vi "Create Missing Source Folders.vi"(8 "error in":errorcluster, 9 "Install Root":string, 10 "Source Root":string, 11 "All Install Folders":path[](array[path])) -> (0 "error out":errorcluster, 1 "Install Root":string, 2 "Source Root":string)   [LabVIEW 2011, in "LVH-Build-Tools.lvlib"]
doc: "This VI creates folders in the source directory to match the folder hierarchy in the install directory."
uses:
  LVH-Build-Tools.lvlib
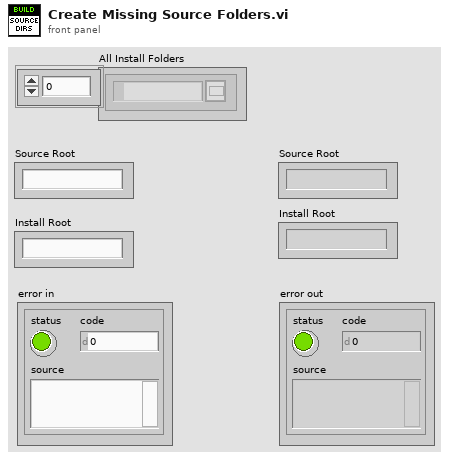
[diagram p1: front panel]
types:
  T1 = typedef "LVH-Build-Tools.lvlib/Configuration.ctl" = cluster{"Source Root":string, "Install Root":string, "Components":string[], "Ignore":string[]}
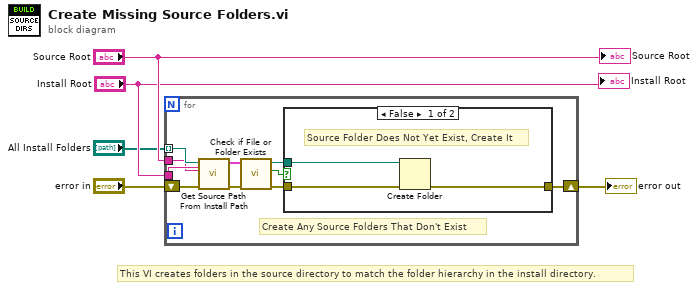
[diagram p0: block diagram]
diagram:
  # "This VI creates folders in the source directory to match the folder hierarchy in the install directory."
  n1 = for {
    tunnel: "All Install Folders" -> [w10] mode=indexing
    shift-right: [w12] -> w3
    shift-left: "error in" -> [w8]
    tunnel: "Install Root" -> [w7]
    tunnel: "Source Root" -> [w6]
    # "Create Any Source Folders That Don't Exist"
    n2 = call "Get Source Path From Install Path.vi"("Error In"=w8, 9:w7, "Install File Path"=w6, "Configuration"=w10) -> ("Error Out"=w9:errorcluster, "Configuraiton"=w11:T1)  [unwired: 4 in, 2 out]
    n3 = call <vilib>:"Check if File or Folder Exists.vi"("error in (no error)"=w9, "path"=w11) -> ("error out"=w13:errorcluster, "file or folder exists?"=w15:bool, "dup path"=w14:path)  [unwired: 7 in]
    n4 = case shown="False" w15 {
      tunnel: w14 -> [w16 _]
      tunnel: w13 -> [w18 w19]
      tunnel: [w17 w19] -> w12
      frame False {
        # "Source Folder Does Not Yet Exist, Create It"
        n5 = Create Folder(path (use dialog)=w16, error in=w18) -> (error out=w17:errorcluster)  [unwired: 1 in, 2 out]
      }
      frame True {
        # "Source Folder Already Exists"
      }
    }
  }
  "error out" <- w3
  "Source Root" <- "Source Root"
  "Install Root" <- "Install Root"
